vi "PluginManager.vi"() -> ()   [LabVIEW 2018]
doc: "This is the central application/framework that controls module, run scripts, etc"
uses:
  LV_Config_class/Config.lvclass/Config.ctl
  Tree/Controls/Plugins Tree Item Type.ctl
  UserEvents/clUserEventDataType.ctl
  LV_Config_class/Accessors/Read ConfigFilePath.vi
  LV_Config_class/Accessors/Write ConfigFilePath.vi
  <vilib>/Utility/error.llb/Error Cluster From Error Code.vi
  <vilib>/ErrorRing/Error Ring.xnode
  Queue/Queue.lvlib
  <userlib>/NIST/NISTErrorLib/NISTErrorLib.lvlib
  LV_Config_class/Config.lvclass
  <vilib>/Utility/config.llb/NI_LVConfig.lvlib
  Message Queue/Message Queue.lvlib
panel:
  out "found?":bool
  in  "Stop?":bool
  out "OrigPluginTreeTags":string[](array[string])
  out "Plugin Tree Caption":string="Available Plugins"
  in  "btnRunModule":bool
  in  "btnRefresh":bool
  in  "btnLoadUserFiles":bool
  in  "btnConfig":bool
  in  "btnAddToTest":bool
  in  "PluginTree":string(tree)
  in  "Experiment Specific Controls":T1(tab)
  in  "Priority":u8=2
  in  "Severity":string="Abort"
  out "Error Out":errorcluster
  in  "Severity":string
  in  "Priority":u8=2
  in  "Create Error (Test AutoTimeout)":bool
  in  "Error In 2":errorcluster
  in  "btnRunScript":bool
  out "Userfiles Folder":path
  in  "btnSaveINIFiles":bool
  in  "btnDeleteScript":bool
  in  "btnNewScript":bool
  in  "btnScriptHelper":bool
  in  "PluginScript":string
  # "Script Preview and Editor"
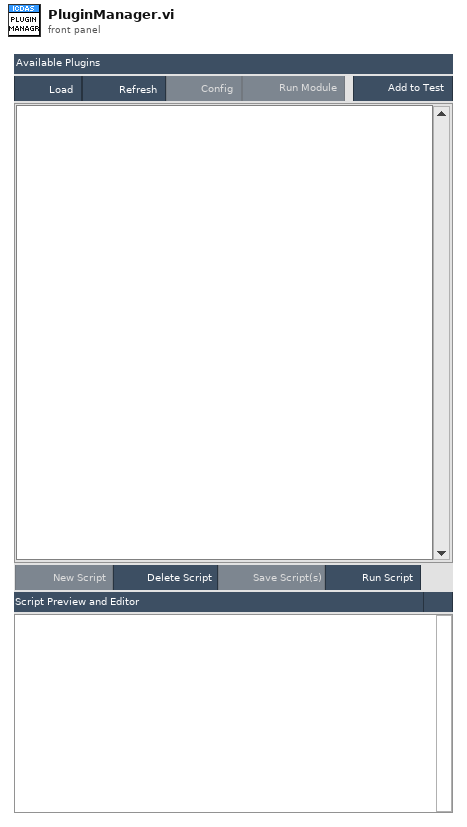
[diagram p1: front panel]
types:
  T1 = enum32{"PV Aging Experiment", "Pacific Power ", "Miscellaneous ", "Errors", "Test AutoTimeout", "Test Python MutliRun"}
  T2 = typedef "ICDASUserEvents.ctl" = cluster{"StopEvent":refnum<user-event>, "RefreshUserEvents":refnum<user-event>, "StatusUpdate":refnum<user-event>, "RunAllScripts":refnum<user-event>, "ShutdownEvent":refnum<user-event>, "TestMgrDidStop":refnum<user-event>, "PluginMgrDidStop":refnum<user-event>}
  T3 = typedef "Message Queue.lvlib/All Message Queues.ctl" = cluster{"UI":refnum<queue>}
  T4 = enum8{"Enabled", "Disabled", "Disabled and Grayed Out"}
  T5 = typedef "Plugins Tree Item Type.ctl" = enum16{"Plugin", "Instrument", "INI File", "INI Script"}
  T6 = typedef "cntlRefs.ctl" = cluster{"rngFGen":refnum<vi>, "rngDigitizer":refnum<vi>, "btnHide":refnum<vi>, "rngInst":refnum<vi>, "PluginTree":refnum<vi>, "TestListboxRef":refnum<vi>, "path.tstFile":refnum<vi>, "cmbxRunningModules":refnum<vi>, "TestDataSubPanel":refnum<vi>, "TestDataCaption":refnum<vi>, "btnPopInOut":refnum<vi>, "PluginMgrQ":refnum<queue>, "TestMgrQ":refnum<queue>, "TestMgrSubPanel":refnum<vi>, "PluginMgrSubPanel":refnum<vi>, "PwrReqHandle":u32, "btnStopOneTest":refnum<vi>, "pathUserfiles":refnum<vi>, "PluginTreeCaption":refnum<vi>, "MainVIRef":refnum<vi>, "btnStatus":refnum<vi>}
  T7 = typedef "NI_LVConfig.lvlib/Config Data RefNum.ctl" = refnum<k1>
  T8 = typedef "Plugin Tree Tag.ctl" = cluster{"ItemType":T5, "Name":string, "Path":path, "Script":string[]}
  T9 = typedef "INIInfo.ctl" = cluster{"Module Name":string, "INI File Name":string, "Class Name":string, "INI File Name Without Extension":string, "Module.Class.INI File Name":string, "Visualization VI Path":path, "Instrument Class Path":path}
  T10 = enum16{"Left Button", "Center Button", "Right Button", "Window Close"}
  T11 = enum32{"Invalid", "Standard", "Closed", "Hidden", "Minimized", "Maximized"}
  T12 = typedef "LVPoint32TypeDef.ctl" = cluster{"Horizontal":i32, "Vertical":i32}
  T13 = typedef "clUserEventDataType.ctl" = cluster{"Data":variant}
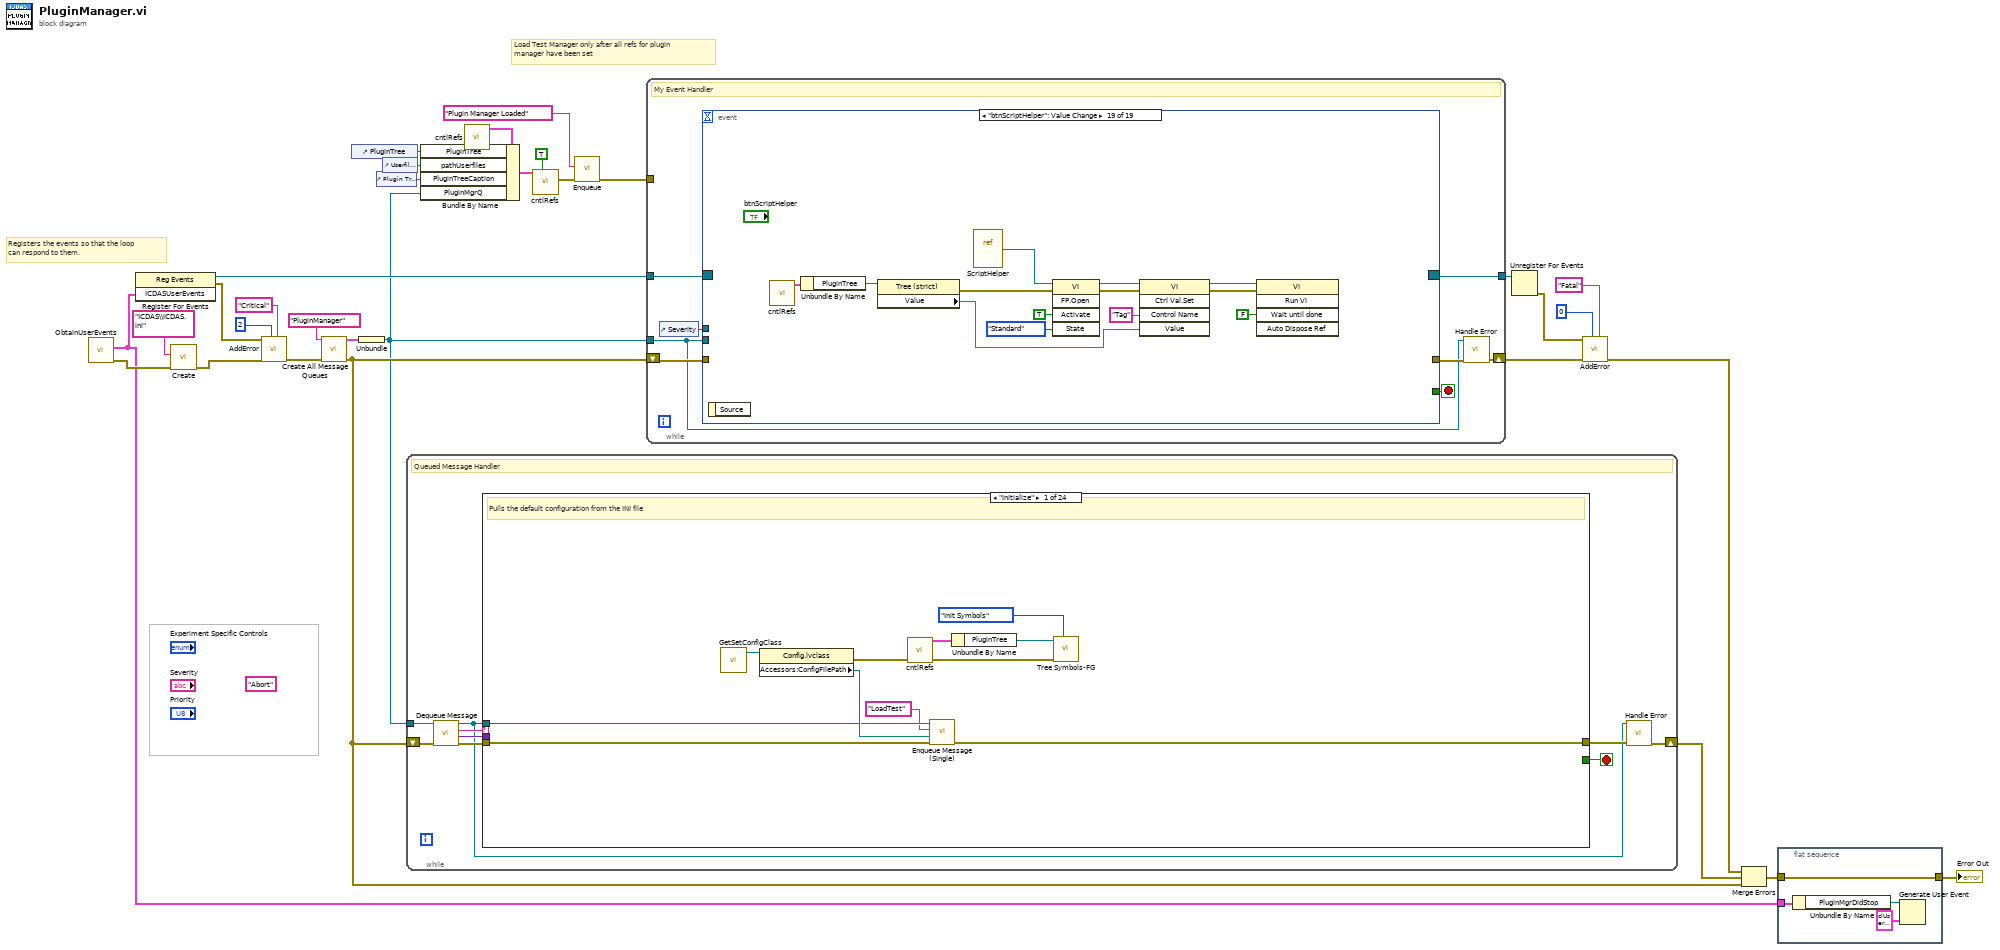
[diagram p0: block diagram]
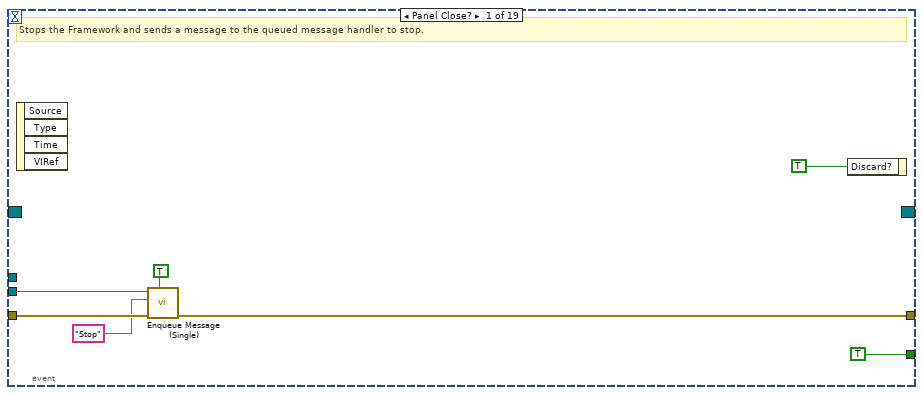
[diagram p2: hidden frame]
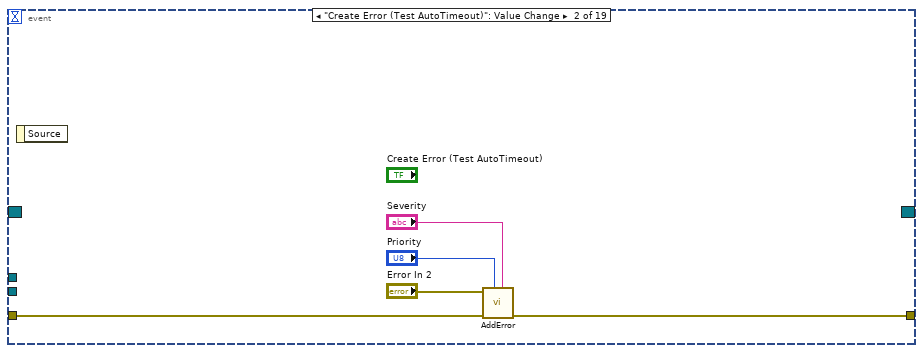
[diagram p3: hidden frame]
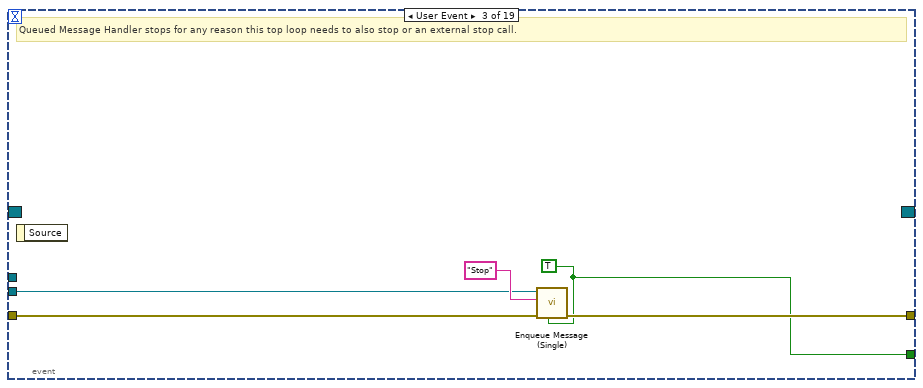
[diagram p4: hidden frame]
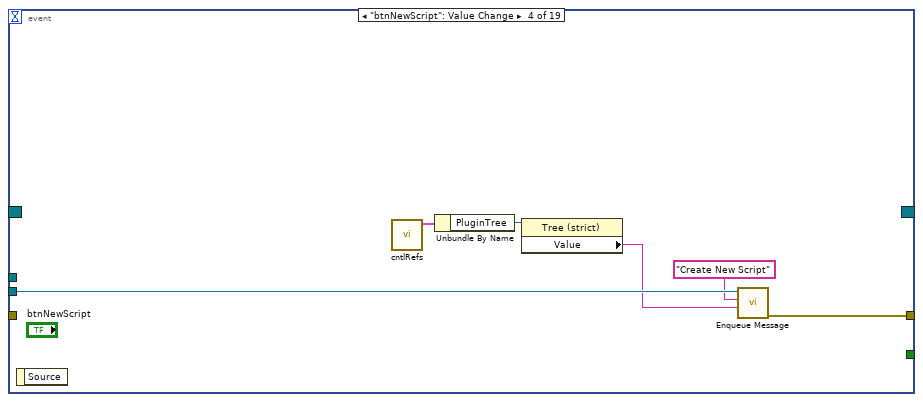
[diagram p5: hidden frame]
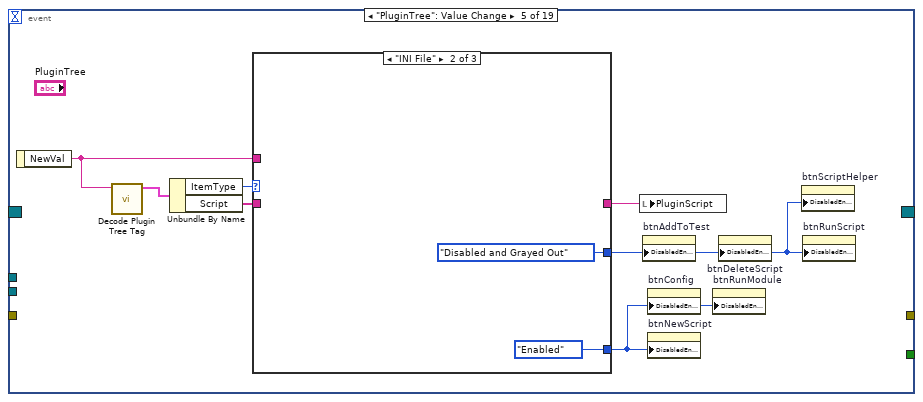
[diagram p6: hidden frame]
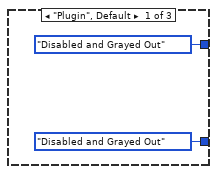
[diagram p7: hidden frame]
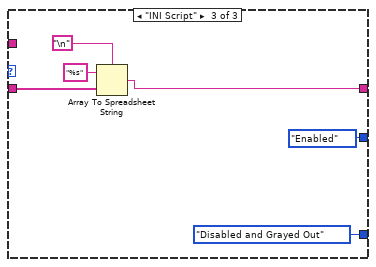
[diagram p8: hidden frame]
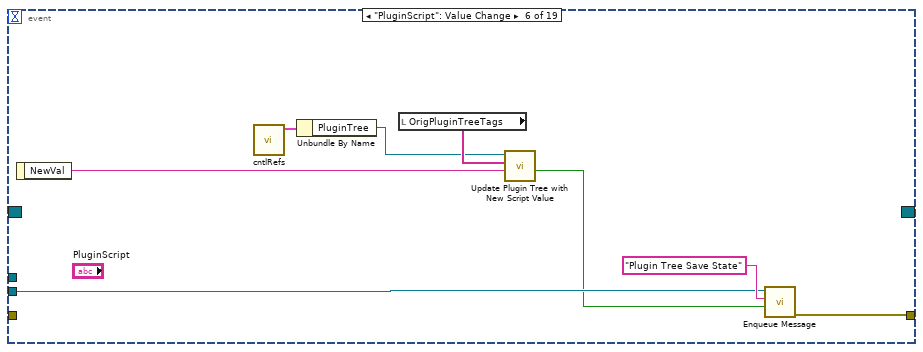
[diagram p9: hidden frame]
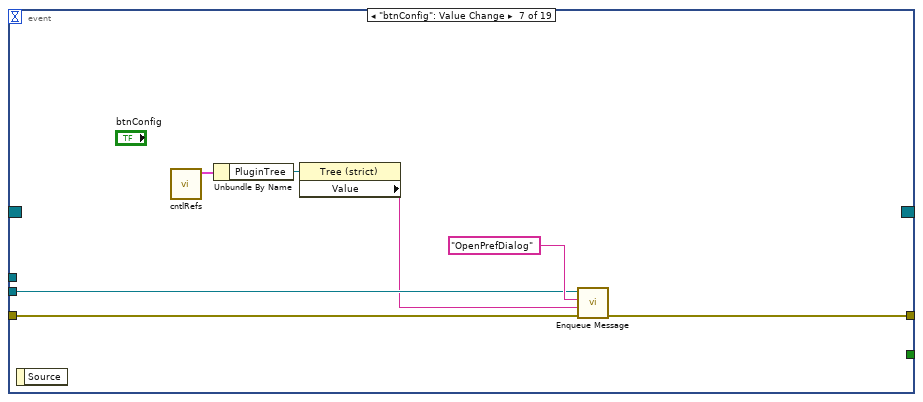
[diagram p10: hidden frame]
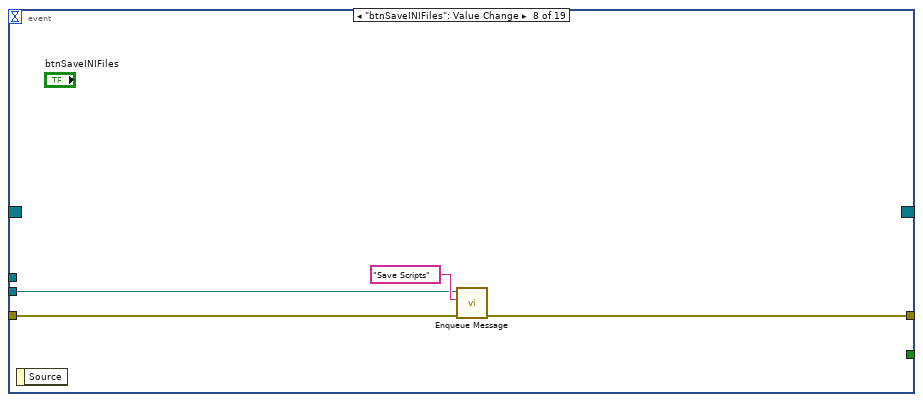
[diagram p11: hidden frame]
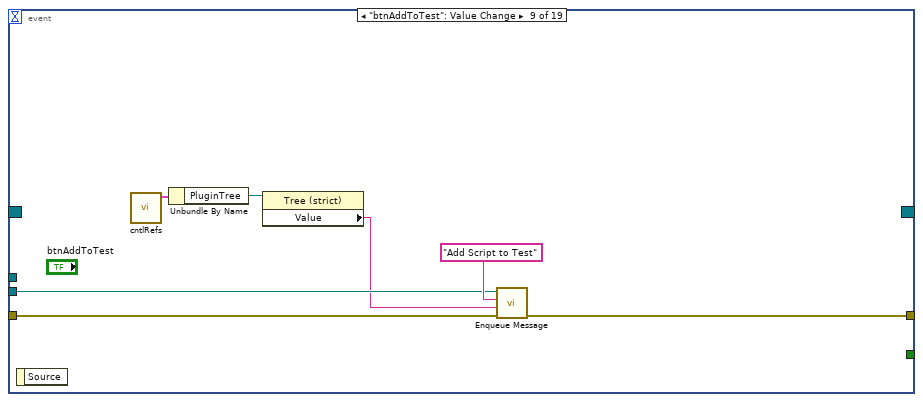
[diagram p12: hidden frame]
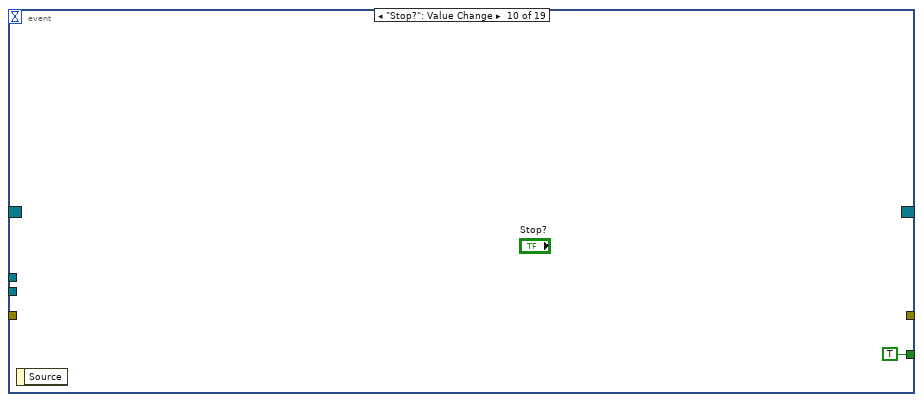
[diagram p13: hidden frame]
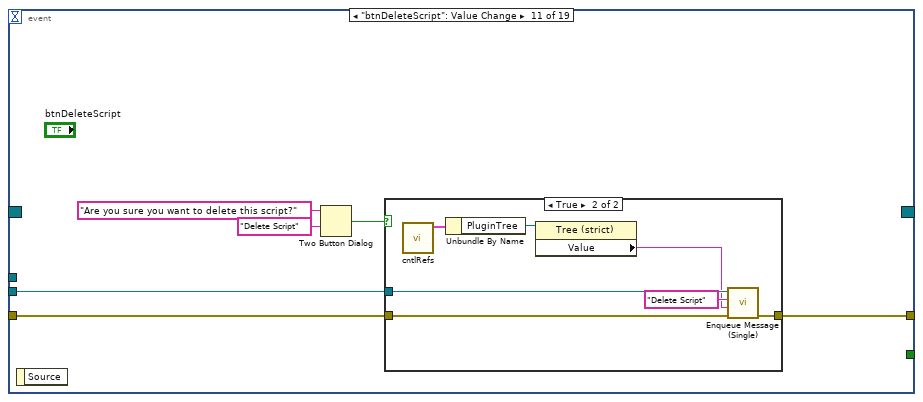
[diagram p14: hidden frame]
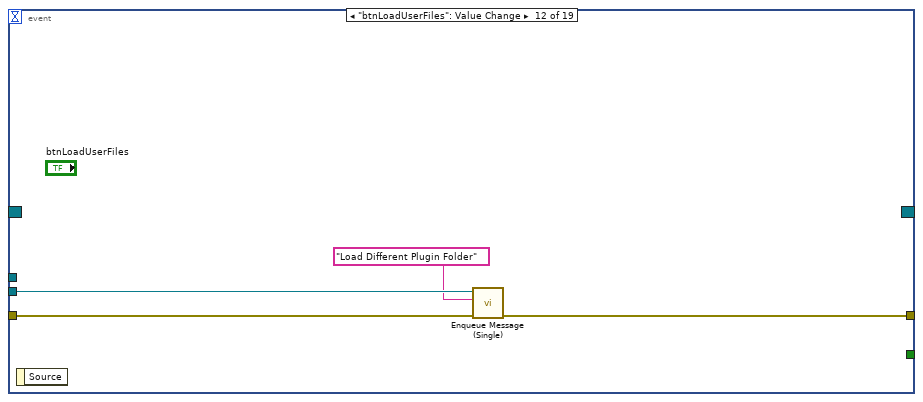
[diagram p16: hidden frame]
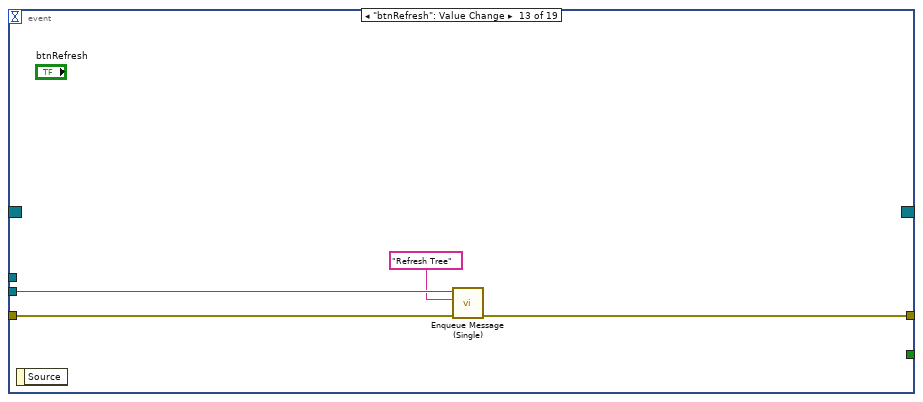
[diagram p17: hidden frame]
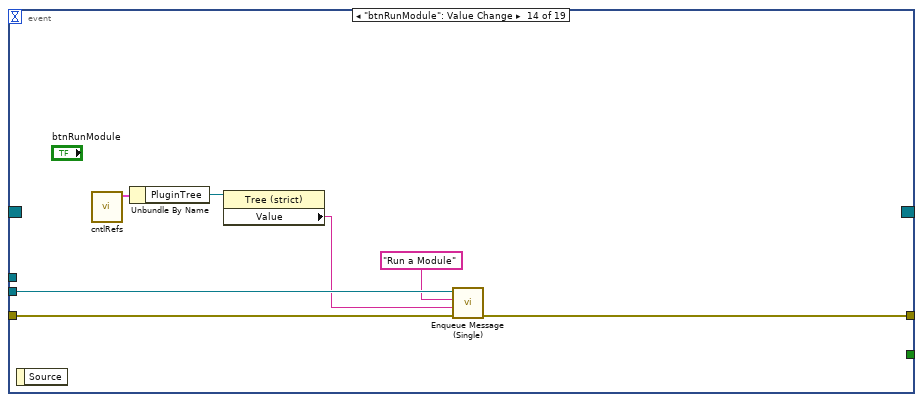
[diagram p18: hidden frame]
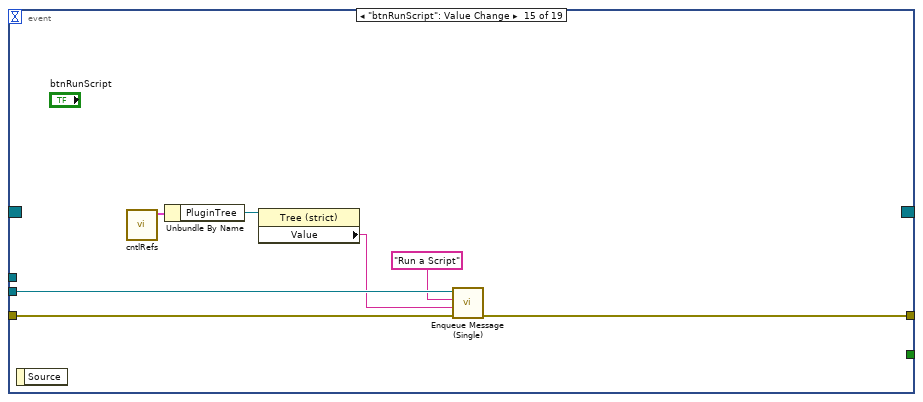
[diagram p19: hidden frame]
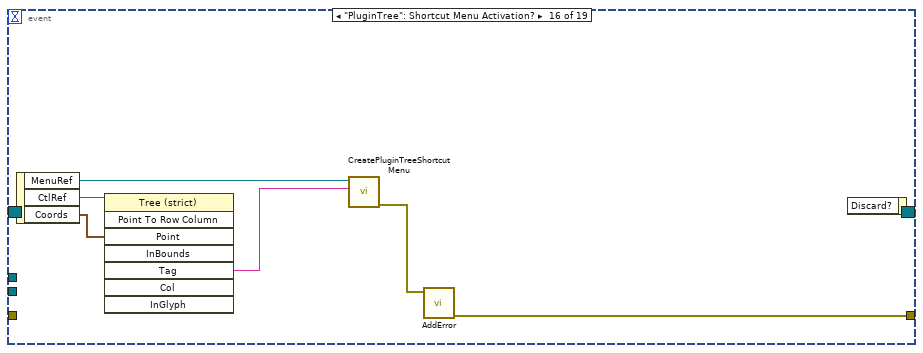
[diagram p20: hidden frame]
diagram:
  (unwired) "Abort" ("Severity")
  # "Load Test Manager only after all refs for plugin\nmanager have been set"
  # "Registers the events so that the loop \ncan respond to them."
  n1 = call "ObtainUserEvents.vi"() -> ("ErrorArray"=w16:errorcluster[], "ICDASUserEvents"=w1:T2)  [unwired: 10 in]
  n2 = register-events(w1) -> (reference out=w31:refnum<event-registration>, error out=w22:errorcluster)  [unwired: 2 in]
  n3 = call "Create.vi"("ErrorArray"=w16, "name or relative path"="ICDAS\\ICDAS.ini") -> ("ErrorArray"=w15:errorcluster[])  [unwired: 8 in, 1 out]
  n4 = call <userlib>:"AddError.vi"("Severity"="Critical", "Priority"=u8 2, "ErrorArray In"=w15, "error in (no error)"=w22) -> ("ErrorArray Out"=w18:errorcluster[])  [unwired: 6 in, 1 out]
  n5 = call "Create All Message Queues.vi"("error in (no error)"=w18, "Queue Name (unnamed)"="PluginManager") -> ("error out"=w9:errorcluster[], "Message Queues out"=w19:T3)  [unwired: 8 in]
  n6 = control-ref of="PluginTree"() -> (w21:refnum<vi>)
  n7 = Unbundle(w19) -> ("UI"=w8:refnum<queue>)
  n8 = control-ref of="Plugin Tree Caption"() -> (w6:refnum<vi>)
  n9 = control-ref of="Userfiles Folder"() -> (w7:refnum<vi>)
  n10 = while {
    shift-right: [w39] -> w27
    shift-left: w9 -> [w34]
    tunnel: w8 -> [w37]
    stop <- w38 stop-if-true
    # "Queued Message Handler"
    n11 = call "Dequeue Message.vi"("error in (no error)"=w34, "Message Queue"=w37) -> ("error out"=w33:errorcluster[], "Message Data"=w36:variant, "Message"=w35:string, "dup Message Queue"=w32:refnum<queue>)  [unwired: 6 in]
    n12 = case shown="\"Initialize\"" w35 {
      selector: w35 -> [_ _ _ _ _ _ w202 _ _ _ _ _ _ _ _ _ _ _ _ _ _ _ _ _]
      tunnel: [w42 w54 w95 w139 w183 w192 w201 w210 w217 w240 w245 w284 w290 w310 w325 w372 w383 w428 w438 w455 w463 w477 w481 w485] -> w40
      tunnel: w33 -> [w44 w53 w100 w138 w178 w196 w200 w210 w223 w240 w247 w284 w302 w314 w319 w374 w384 w428 w437 w454 w464 w477 w481 w485]
      tunnel: [_ _ _ _ _ TRUE _ _ _ _ _ _ _ _ _ _ _ _ _ _ _ _ _ _] -> w38
      tunnel: w36 -> [_ w52 w101 _ w182 _ _ _ w213 w238 w244 w268 w294 w308 _ _ _ _ w432 w449 w461 _ _ _]
      tunnel: w32 -> [w43 w51 w93 w129 w173 w187 _ _ w216 _ w246 _ _ _ w320 w371 w385 _ _ _ _ _ _ _]
      frame "Initialize" {
        # "Pulls the default configuration from the INI file"
        n13 = call "GetSetConfigClass.vi"() -> ("Ref out"=w50:refnum<class "Config.lvclass">)  [unwired: 11 in]
        n14 = property class="Config.lvclass"(reference=w50) -> (error out=w47:errorcluster, "Accessors:ConfigFilePath"=w49:path)  [unwired: 1 in, 1 out]
        n15 = call "cntlRefs.vi"() -> ("cntlRefs"=w46:T6)  [unwired: 10 in, 1 out]
        n16 = call "Enqueue Message (Single).vi"("error in (no error)"=w44, "Message Data"=w49, "Message"="LoadTest", "Message Queue"=w43) -> ("error out"=w42:errorcluster[])  [unwired: 6 in, 1 out]
        n17 = Unbundle By Name(w46) -> ("PluginTree"=w45:refnum<vi>)
        n18 = call "Tree Symbols-FG.vi"("Actions"=enum16{"Init Symbols", "Set Item Symbol"}."Init Symbols", "error in (no error)"=w47, "Tree Ref"=w45) -> ()  [unwired: 5 in, 4 out]
      }
      frame "LoadTest" {
        # "From the default file load the last saved results and updated the controls and indicators"
        n19 = disable-structure shown="Enabled" {
          disable-tunnel: [w87 _] -> w54
          disable-tunnel: w53 -> [w85 _]
          disable-tunnel: w52 -> [w82 w88]
          disable-tunnel: w51 -> [w66 _]
          frame Enabled {
            n20 = call "cntlRefs.vi"() -> ("cntlRefs"=w59:T6)  [unwired: 10 in, 1 out]
            n21 = Unbundle By Name(w59) -> ("pathUserfiles"=w58:refnum<vi>)
            n22 = Variant To Data(type=path "", Variant=w82) -> (data=w83:path, error out=w86:errorcluster)  [unwired: 1 in]
            n23 = call <vilib>:"Open Config Data.vi"("error in (no error)"=w86, "configuration file path"=w83) -> ("error out"=w67:errorcluster, "refnum"=w81:T7)  [unwired: 7 in, 1 out]
            n24 = property class="Path"(reference=w58, error in=w67) -> (error out=w78:errorcluster, "Label.Text"=w79:string)  [unwired: 1 out]
            n25 = call <userlib>:"Read Key (Variant)__ogtk.vi"("section"=w79, "error in (no error)"=w78, "type"="", "key (optional)"=w79, "refnum"=w81) -> ("error out"=w77:errorcluster, "key-value"=w80:variant, "found?"=→"found?":bool)  [unwired: 3 in, 1 out]
            n26 = Variant To Data(error in=w77, type="", Variant=w80) -> (data=w76:string, error out=w73:errorcluster)
            n27 = call <vilib>:"Trim Whitespace.vi"("string"=w76) -> ("trimmed string"=w71:string)  [unwired: 1 in]
            n28 = local read "Severity"() -> (w74:string)
            n29 = local read "Priority"() -> (w75:u8)
            n30 = call <vilib>:"Application Directory.vi"() -> ("Application Directory"=w61:path)
            n31 = Empty String/Path?(string/path=w71) -> (empty?=w70:bool)
            n32 = call <userlib>:"AddError.vi"("Severity"=w74, "Priority"=w75, "ErrorArray In"=w85, "error in (no error)"=w73) -> ("ErrorArray Out"=w64:errorcluster[])  [unwired: 6 in, 1 out]
            n33 = Build Path(base path=w61, name or relative path=w71) -> (appended path=w69:path)
            n34 = Build Path(base path=w61, name or relative path="UserFiles") -> (appended path=w60:path)
            n35 = Select(t=w60, s=w70, f=w69) -> (s? t:f=w68:path)
            n36 = call "Enqueue Defer Panel Updates Message.vi"("error in (no error)"=w64, "Message Queue"=w66) -> ("error out"=w63:errorcluster[], "dup Message Queue"=w65:refnum<queue>)  [unwired: 8 in]
            n37 = call "Enqueue Message (Single).vi"("error in (no error)"=w63, "Message Data"=w68, "Message"="Populate Plugin Tree", "Message Queue"=w65) -> ("error out"=w87:errorcluster[])  [unwired: 6 in, 1 out]
          }
          frame Disabled {
            n38 = disable-structure shown="Disabled" {
              disable-tunnel: w88 -> [w90 _]
              frame Disabled {
                n39 = Variant To Data(type=path "", Variant=w90) -> (data=w91:path, error out=w89:errorcluster)  [unwired: 1 in]
                n40 = call <vilib>:"Open Config Data.vi"("error in (no error)"=w89, "configuration file path"=w91) -> ()  [unwired: 7 in, 3 out]
              }
              frame Enabled {
              }
            }
          }
        }
      }
      frame "Error" {
        n41 = Variant To Data(type=w100, Variant=w101) -> (data=w99:errorcluster[], error out=w94:errorcluster)  [unwired: 1 in]
        n42 = call <userlib>:"ParseErrors.vi"("ErrorArray"=w99) -> ("ErrorArray"=w102:errorcluster[])  [unwired: 8 in, 2 out]
        n43 = for {
          tunnel: w102 -> [w109] mode=indexing
          tunnel: [w112] -> w96 mode=concatenating
          tunnel: w93 -> [w103]
          n44 = call <userlib>:"GeneralHandler.vi"("error in (no error)"=w109) -> ("Severity"=w110:string, "Stop"=w106:bool, "Abort"=w107:bool, "Continue"=w108:bool, "Error Out"=w104:errorcluster)  [unwired: 6 in]
          n45 = Build Array(w108, w107, w106) -> (w105:bool[])
          n46 = Boolean Array To Number(Boolean array=w105) -> (number=w111:u32)
          n47 = case shown="2" w111 {
            tunnel: w110 -> [_ _ _ _]
            tunnel: [_ _ w115 w128] -> w112
            tunnel: w109 -> [_ _ _ _]
            tunnel: w104 -> [_ _ w117 _]
            tunnel: w103 -> [_ _ w114 _]
            frame 0, Default {
              # "No Dialog"
            }
            frame 1 {
              # "Continue"
            }
            frame 2 {
              # "Abort Button Pressed"
              n48 = Flush Queue(queue=w114, error in (no error)=w117) -> (queue out=w113:refnum<queue>, error out=w120:errorcluster)  [unwired: 1 out]
              n49 = call <userlib>:"AddError.vi"("Severity"="Critical", "Priority"=u8 1, "error in (no error)"=w120) -> ("ErrorArray Out"=w116:errorcluster[])  [unwired: 7 in, 1 out]
              n50 = disable-structure shown="Disabled" {
                disable-tunnel: w116 -> [w124 w127]
                disable-tunnel: [w123 w127] -> w115
                disable-tunnel: w113 -> [w121 _]
                frame Disabled {
                  n51 = To Variant(anything="*AbortScript" ("Message")) -> (Variant=w125:variant)
                  n52 = call-poly "Enqueue Message.vi"("error in (no error)"=w124, "Message Data"=w125, "Message"="RunOneTest", "Message Queue"=w121) -> ("error out"=w123:errorcluster[])  [unwired: 6 in, 1 out]
                }
                frame Enabled {
                }
              }
            }
            frame 4 {
              # "Stop this application"
              n53 = call "StopEvent.vi"() -> ("ErrorArray"=w128:errorcluster[])  [unwired: 11 in]
            }
          }
        }
        n54 = call <userlib>:"AddError.vi"("Severity"="Fatal", "Priority"=u8 0, "ErrorArray In"=w96, "error in (no error)"=w94) -> ("ErrorArray Out"=w95:errorcluster[])  [unwired: 6 in, 1 out]
      }
      frame "Stop" {
        n55 = disable-structure shown="Enabled" {
          disable-tunnel: [w158 FALSE ("T button?")] -> w134
          frame Disabled {
            n56 = Two Button Dialog(message="Save Application configuration to a new location?") -> (T button?=w158:bool)  [unwired: 2 in]
          }
          frame Enabled {
          }
        }
        n57 = call "GetSetConfigClass.vi"() -> ("Ref out"=w142:refnum<class "Config.lvclass">)  [unwired: 11 in]
        n58 = property class="Config.lvclass"(reference=w142) -> (reference out=w132:refnum<class "Config.lvclass">, error out=w135:errorcluster, "Accessors:ConfigFilePath"=w136:path)  [unwired: 1 in]
        n59 = case shown="True" w134 {
          tunnel: w136 -> [w143 w154]
          tunnel: w135 -> [w144 w153]
          tunnel: [w144 w145] -> w133
          tunnel: w132 -> [_ w149]
          tunnel: [w143 w146] -> w131
          frame False {
          }
          frame True {
            n60 = call "FileDialog.vi"("Error In"=w153, "File Path Control In"=w154) -> ("Error Out"=w151:errorcluster, "Valid File Path?"=w148:bool, "File Path Control Out"=w147:path)  [unwired: 7 in]
            n61 = Select(t=w147, s=w148, f=w154) -> (s? t:f=w152:path)
            n62 = property class="Config.lvclass"(reference=w149, error in=w151, "Accessors:ConfigFilePath"=w152) -> (reference out=w150:refnum<class "Config.lvclass">, error out=w145:errorcluster, "Accessors:ConfigFilePath"=w146:path)
            n63 = flat-sequence {
              tunnel: w150 -> [w157]
              tunnel: w145 -> [_]
              frame #0 {
                n64 = Two Button Dialog(message="Update configuration file path") -> (T button?=w156:bool)  [unwired: 2 in]
                n65 = call "GetSetConfigClass.vi"("Set (f)"=w156, "Ref in"=w157) -> ()  [unwired: 9 in, 1 out]
              }
            }
          }
        }
        n66 = local read "Severity"() -> (w130:string)
        n67 = call-poly "Enqueue Message.vi"("error in (no error)"=w138, "Message Data"=w131, "Message"="SaveTest", "Message Queue"=w129) -> ("error out"=w137:errorcluster[])  [unwired: 6 in, 1 out]
        n68 = call <userlib>:"AddError.vi"("Severity"=w130, "Priority"=u8 0, "ErrorArray In"=w137, "error in (no error)"=w133) -> ("ErrorArray Out"=w139:errorcluster[])  [unwired: 6 in, 1 out]
      }
      frame "SaveTest" {
        # "saves the state of the controls and indicators into an INI file"
        n69 = Variant To Data(type=path "", Variant=w182) -> (data=w177:path, error out=w181:errorcluster)  [unwired: 1 in]
        n70 = call <vilib>:"Open Config Data.vi"("error in (no error)"=w181, "configuration file path"=w177) -> ("error out"=w180:errorcluster, "refnum"=w176:T7)  [unwired: 7 in, 1 out]
        n71 = call <userlib>:"AddError.vi"("ErrorArray In"=w178, "error in (no error)"=w180) -> ("ErrorArray Out"=w179:errorcluster[])  [unwired: 8 in, 1 out]
        n72 = call "cntlRefs.vi"() -> ("cntlRefs"=w174:T6)  [unwired: 10 in, 1 out]
        n73 = Unbundle By Name(w174) -> ("pathUserfiles"=w170:refnum<vi>)
        n74 = property class="Path"(reference=w170) -> (error out=w166:errorcluster, "Label.Text"=w167:string, "Value"=w165:path)  [unwired: 1 in, 1 out]
        n75 = call "ConvertAbsolutePathToRelative.vi"("Absolute Path"=w165) -> ("RelativePath"=w164:string)  [unwired: 10 in]
        n76 = call <userlib>:"Write Key (Variant)__ogtk.vi"("section"=w167, "error in (no error)"=w166, "key-value"=w164, "key (optional)"=w167, "refnum"=w176) -> ("error out"=w163:errorcluster, "refnum out"=w161:T7)  [unwired: 5 in]
        n77 = call <vilib>:"Close Config Data.vi"("error in (no error)"=w163, "refnum"=w161) -> ("error out"=w162:errorcluster)  [unwired: 8 in, 1 out]
        n78 = call <userlib>:"AddError.vi"("Severity"="Abort", "Priority"=u8 3, "ErrorArray In"=w179, "error in (no error)"=w162) -> ("ErrorArray Out"=w171:errorcluster[])  [unwired: 6 in, 1 out]
        n79 = call-poly "Enqueue Message.vi"("error in (no error)"=w171, "Message"="End", "Message Queue"=w173) -> ("error out"=w183:errorcluster[])  [unwired: 7 in, 1 out]
      }
      frame "End" {
        n80 = call "cntlRefs.vi"() -> ("cntlRefs"=w191:T6)  [unwired: 10 in, 1 out]
        n81 = Unbundle By Name(w191) -> ("PluginTree"=w190:refnum<vi>)
        n82 = local write "PluginScript"("") -> ()
        n83 = invoke class="Tree (strict)" method="Edit Tree Items.Delete"(reference=w190, "Delete Children"=TRUE ("Delete Children?")) -> ()  [unwired: 3 in, 5 out]
        n84 = Release Queue(queue=w187, force destroy? (F)=TRUE) -> (error out=w186:errorcluster)  [unwired: 1 in, 2 out]
        n85 = property on="Stop?" class="Bool (strict)"("Val(Sgnl)"=TRUE ("Value (Signaling)")) -> ()  [unwired: 2 in, 2 out]
        n86 = call <userlib>:"AddError.vi"("Severity"="Abort", "Priority"=u8 3, "ErrorArray In"=w196, "error in (no error)"=w186) -> ("ErrorArray Out"=w192:errorcluster[])  [unwired: 6 in, 1 out]
      }
      frame Default {
        n87 = xnode "Error Ring"("parameter 0"=w202) -> ("error out"=w197:errorcluster)
        n88 = call <userlib>:"AddError.vi"("Severity"="Inform", "Priority"=u8 5, "ErrorArray In"=w200, "error in (no error)"=w197) -> ("ErrorArray Out"=w201:errorcluster[])  [unwired: 6 in, 1 out]
      }
      frame "----Plugin Setup----" {
      }
      frame "Populate Plugin Tree" {
        # "Clear tree value and script control"
        n89 = Variant To Data(type=path "", Variant=w213) -> (data=w211:path)  [unwired: 1 in, 1 out]
        "Userfiles Folder" <- w211
        n90 = call "cntlRefs.vi"() -> ("cntlRefs"=w215:T6)  [unwired: 10 in, 1 out]
        n91 = Unbundle By Name(w215) -> ("PluginTree"=w214:refnum<vi>)
        n92 = call "Populate Plugin Tree.vi"("ErrorArray In"=w223, "Userfiles Directory"=w211, "PluginTreeRef"=w214) -> ("ErrorArray Out"=w218:errorcluster[], "All Tags"=→"OrigPluginTreeTags":string[], "Tree Ref out"=w225:refnum<vi>)  [unwired: 5 in, 1 out]
        n93 = property class="Tree (strict)"(reference=w225, "Val(Sgnl)"="") -> ()  [unwired: 1 in, 2 out]
        n94 = call "Enqueue Message (Single).vi"("error in (no error)"=w218, "Message Data"=FALSE, "Message"="Plugin Tree Save State", "Message Queue"=w216) -> ("error out"=w222:errorcluster[], "dup Message Queue"=w221:refnum<queue>)  [unwired: 6 in]
        n95 = call "Enqueue Update Panel Message.vi"("error in (no error)"=w222, "Message Queue"=w221) -> ("error out"=w217:errorcluster[])  [unwired: 8 in, 1 out]
      }
      frame "Plugin Tree Save State" {
        n96 = Variant To Data(type=FALSE, Variant=w238) -> (data=w234:bool)  [unwired: 1 in, 1 out]
        n97 = local read "Userfiles Folder"() -> (w230:path)
        n98 = call "ConvertAbsolutePathToRelative.vi"("Absolute Path"=w230) -> ("RelativePath"=w227:string)  [unwired: 10 in]
        n99 = Format Into String(format string="Available Plugins - %s" ("Message"), w227) -> (resulting string=w228:string)  [unwired: 2 in, 1 out]
        n100 = Concatenate Strings(w228, "*" ("string")) -> (w236:string)
        n101 = Select(t=w236, s=w234, f=w228) -> (s? t:f=→"Plugin Tree Caption":string)
        n102 = Select(t=T4."Enabled" ("Disabled"), s=w234, f=T4."Disabled and Grayed Out" ("Disabled")) -> (s? t:f=w232:T4)
        n103 = property on="btnSaveINIFiles" class="Bool"("DisabledEnum"=w232) -> ()  [unwired: 2 in, 2 out]
      }
      frame "Create New Script" {
        n104 = Variant To Data(type="", Variant=w244) -> (data=w242:string, error out=w241:errorcluster)  [unwired: 1 in]
        n105 = call "cntlRefs.vi"() -> ("cntlRefs"=w252:T6)  [unwired: 10 in, 1 out]
        n106 = call "Decode Plugin Tree Tag.vi"("error in (no error)"=w241, "Tag"=w242) -> ("error out"=w250:errorcluster, "Plugin Tree Tag"=w248:T8)  [unwired: 8 in]
        n107 = Unbundle By Name(w252) -> ("PluginTree"=w251:refnum<vi>)
        n108 = Unbundle By Name(w248) -> ("ItemType"=w249:T5)
        n109 = case shown="\"INI File\"" w249 {
          tunnel: w251 -> [_ w261]
          tunnel: w250 -> [_ w259]
          tunnel: w242 -> [_ w260]
          tunnel: w246 -> [_ w256]
          tunnel: [w253 w255] -> w245
          tunnel: w247 -> [w253 w254]
          frame "Plugin", Default {
          }
          frame "INI File" {
            n110 = call "Add New Script to Tree.vi"("error in (no error)"=w259, "Value"=w260, "TreeControl in"=w261) -> ("error out"=w257:errorcluster, "Cancelled?"=w258:bool)  [unwired: 7 in]
            n111 = case shown="False" w258 {
              tunnel: w257 -> [_ _]
              tunnel: w256 -> [w264 _]
              tunnel: [w263 _] -> w255
              tunnel: w254 -> [w262 _]
              frame False {
                n112 = call-poly "Enqueue Message.vi"("error in (no error)"=w262, "Message Data"=TRUE, "Message"="Plugin Tree Save State", "Message Queue"=w264) -> ("error out"=w263:errorcluster[])  [unwired: 6 in, 1 out]
              }
              frame True {
              }
            }
          }
        }
      }
      frame "Delete Script" {
        n113 = Variant To Data(type="", Variant=w268) -> (data=w267:string)  [unwired: 1 in, 1 out]
        n114 = call "cntlRefs.vi"() -> ("cntlRefs"=w283:T6)  [unwired: 10 in, 1 out]
        n115 = Unbundle By Name(w283) -> ("PluginTree"=w282:refnum<vi>)
        n116 = invoke class="Tree (strict)" method="Edit Tree Items.Delete"(reference=w282, "tag"=w267, "Delete Children"=TRUE ("Delete Children?")) -> (error out=w271:errorcluster)  [unwired: 2 in, 4 out]
        n117 = call "Decode Plugin Tree Tag.vi"("error in (no error)"=w271, "Tag"=w267) -> ("error out"=w273:errorcluster, "Plugin Tree Tag"=w281:T8)  [unwired: 8 in]
        n118 = Unbundle By Name(w281) -> ("Name"=w275:string, "Path"=w280:path)
        n119 = call <vilib>:"Open Config Data.vi"("error in (no error)"=w273, "configuration file path"=w280) -> ("error out"=w278:errorcluster, "refnum"=w279:T7)  [unwired: 7 in, 1 out]
        n120 = Concatenate Strings("*" ("string"), w275) -> (w270:string)
        n121 = call <vilib>:"Remove Section.vi"("section"=w270, "error in (no error)"=w278, "refnum"=w279) -> ("error out"=w276:errorcluster, "refnum out"=w277:T7)  [unwired: 6 in, 1 out]
        n122 = call <vilib>:"Close Config Data.vi"("error in (no error)"=w276, "refnum"=w277) -> ()  [unwired: 8 in, 2 out]
      }
      frame "OpenPrefDialog" {
        # "Get module name from INI File Path"
        # "runs the SSM using a set script"
        n123 = call "cntlRefs.vi"() -> ("cntlRefs"=w288:T6)  [unwired: 10 in, 1 out]
        n124 = Unbundle By Name(w288) -> ("MainVIRef"=w287:refnum<vi>)
        n125 = call <vilib>:"Set Busy.vi"("VI reference (current VI)"=w287) -> ("error out"=w291:errorcluster)  [unwired: 9 in, 1 out]
        n126 = Variant To Data(error in=w291, type="", Variant=w294) -> (data=w293:string, error out=w292:errorcluster)
        n127 = call "Decode Plugin Tree Tag.vi"("error in (no error)"=w292, "Tag"=w293) -> ("error out"=w297:errorcluster, "Plugin Tree Tag"=w301:T8)  [unwired: 8 in]
        n128 = Unbundle By Name(w301) -> ("Path"=w300:path)
        n129 = call <userlib>:"AddError.vi"("Severity"="Inform", "Priority"=u8 2, "ErrorArray In"=w302, "error in (no error)"=w297) -> ("ErrorArray Out"=w296:errorcluster[])  [unwired: 6 in, 1 out]
        n130 = call "ExtractINIInfo.vi"("INI File Path"=w300) -> ("INI Info"=w286:T9)  [unwired: 8 in, 2 out]
        n131 = Unbundle By Name(w286) -> ("Module.Class.INI File Name"=w285:string)
        n132 = call "Load PrefDialog For an INI File.vi"("Error Array In"=w296, "PathToPluginINI"=w300, "Plugin Name"=w285) -> ("ErrorArray Out"=w290:errorcluster[])  [unwired: 8 in]
        n133 = Index Array(array=w290) -> (element=w289:errorcluster)  [unwired: 1 in]
        n134 = call <vilib>:"Unset Busy.vi"("error in (no error)"=w289, "VI reference (current VI)"=w287) -> ()  [unwired: 9 in, 1 out]
      }
      frame "Open in Editor" {
        # "Get module name from INI File Path"
        # "runs the SSM using a set script"
        n135 = Variant To Data(type="", Variant=w308) -> (data=w307:string, error out=w306:errorcluster)  [unwired: 1 in]
        n136 = call "Decode Plugin Tree Tag.vi"("error in (no error)"=w306, "Tag"=w307) -> ("error out"=w304:errorcluster, "Plugin Tree Tag"=w313:T8)  [unwired: 8 in]
        n137 = Unbundle By Name(w313) -> ("Path"=w305:path)
        n138 = call <vilib>:"Open a Document on Disk.vi"("error in (no error)"=w304, "document path"=w305) -> ("error out"=w303:errorcluster)  [unwired: 5 in]
        n139 = call <userlib>:"AddError.vi"("Severity"="Inform", "Priority"=u8 2, "ErrorArray In"=w314, "error in (no error)"=w303) -> ("ErrorArray Out"=w310:errorcluster[])  [unwired: 6 in, 1 out]
      }
      frame "Load Different Plugin Folder" {
        n140 = local read "Plugin Tree Caption"() -> (w324:string)
        n141 = Match Pattern(string=w324, regular expression="*") -> (offset past match=w322:i32)  [unwired: 1 in, 3 out]
        n142 = Greater Than 0?(x=w322) -> (x > 0?=w316:bool)
        n143 = case shown="True" w316 {
          tunnel: "There are unsaved changes in the plugin structure.Please select what you would like to do next." ("message") -> [_ w339]
          tunnel: w320 -> [w327 w333]
          tunnel: w319 -> [w326 w332]
          tunnel: [TRUE ("Allow user to close window? (TRUE)") w331] -> w321
          tunnel: [w327 w330] -> w318
          tunnel: [w326 w329] -> w317
          frame False {
          }
          frame True {
            n144 = call <vilib>:"Three Button Dialog.vi"("Allow user to close window? (TRUE)"=FALSE, "Justify Message (Left)"=enum16{"Left", "Center", "Right"}."Center", "Center Button Text (\"No\")"="Discard Changes & Load" ("Left Button Text (\"Yes\")"), "Left Button Text (\"Yes\")"="Save Changes & Load" ("Left Button Text (\"Yes\")"), "message"=w339) -> ("Which Button?"=w334:T10)  [unwired: 6 in]
            n145 = case shown="\"Left Button\"" w334 {
              tunnel: w333 -> [w343 w347 w350]
              tunnel: w332 -> [w344 w346 w349]
              tunnel: [TRUE ("Allow user to close window? (TRUE)") TRUE ("Allow user to close window? (TRUE)") FALSE ("Allow user to close window? (TRUE)")] -> w331
              tunnel: [w341 w347 w350] -> w330
              tunnel: [w340 w346 w349] -> w329
              frame "Left Button" {
                n146 = call "Enqueue Message (Single).vi"("error in (no error)"=w344, "Message"="Save Scripts", "Message Queue"=w343) -> ("error out"=w340:errorcluster[], "dup Message Queue"=w341:refnum<queue>)  [unwired: 7 in]
              }
              frame "Center Button" {
              }
              frame "Right Button", Default {
              }
            }
          }
        }
        n147 = case shown="True" w321 {
          tunnel: w317 -> [w352 w356]
          tunnel: w318 -> [_ w355]
          tunnel: [w352 w354] -> w325
          frame False {
          }
          frame True {
            n148 = call <vilib>:"Application Directory.vi"() -> ("Application Directory"=w359:path)
            n149 = call "File Dialog"("start path"=w359, "prompt"="Navigate into \"UserFiles\" folder and press \"Select Folder\" button to load...") -> ("selected path"=w353:path, "cancelled"=w357:bool)  [unwired: 10 in, 2 out]
            n150 = case shown="False" w357 {
              tunnel: w356 -> [w362 w367]
              tunnel: w355 -> [w363 _]
              tunnel: [w365 w367] -> w354
              tunnel: w353 -> [w364 _]
              frame False {
                n151 = call "Enqueue Defer Panel Updates Message.vi"("error in (no error)"=w362, "Message Queue"=w363) -> ("error out"=w360:errorcluster[], "dup Message Queue"=w361:refnum<queue>)  [unwired: 8 in]
                n152 = call "Enqueue Message (Single).vi"("error in (no error)"=w360, "Message Data"=w364, "Message"="Populate Plugin Tree", "Message Queue"=w361) -> ("error out"=w365:errorcluster[])  [unwired: 6 in, 1 out]
              }
              frame True {
              }
            }
          }
        }
      }
      frame "Save Scripts" {
        # "After saving the new configuratin, replace the Original Tags\nAND\nRefresh test scrip previoew in Test Manager"
        # "Set tree state to FALSE or already saved"
        n153 = call "cntlRefs.vi"() -> ("cntlRefs"=w380:T6)  [unwired: 10 in, 1 out]
        n154 = Unbundle By Name(w380) -> ("TestMgrQ"=w370:refnum<queue>, "PluginTree"=w379:refnum<vi>)
        n155 = call "Save Plugin Scripts.vi"("TreeControl in"=w379) -> ("error out"=w378:errorcluster, "New Tags After Save"=w377:string[])  [unwired: 8 in, 1 out]
        n156 = property on="OrigPluginTreeTags" class="Arr (strict)"(error in=w378, "Value"=w377) -> (error out=w368:errorcluster)  [unwired: 1 in, 1 out]
        n157 = call-poly "Enqueue Message.vi"("Message"="Refresh Test Script", "Message Queue"=w370) -> ()  [unwired: 8 in, 2 out]
        n158 = call <userlib>:"AddError.vi"("Severity"="Inform", "Priority"=u8 2, "ErrorArray In"=w374, "error in (no error)"=w368) -> ("ErrorArray Out"=w373:errorcluster[])  [unwired: 6 in, 1 out]
        n159 = call-poly "Enqueue Message.vi"("error in (no error)"=w373, "Message Data"=FALSE, "Message"="Plugin Tree Save State", "Message Queue"=w371) -> ("error out"=w372:errorcluster[])  [unwired: 6 in, 1 out]
      }
      frame "Refresh Tree" {
        n160 = local read "Plugin Tree Caption"() -> (w388:string)
        n161 = Match Pattern(string=w388, regular expression="*") -> (offset past match=w386:i32)  [unwired: 1 in, 3 out]
        n162 = Greater Than 0?(x=w386) -> (x > 0?=w389:bool)
        n163 = case shown="True" w389 {
          tunnel: "There are unsaved changes in the plugin structure.Please select what you would like to do next." ("message") -> [_ w407]
          tunnel: w385 -> [w395 w401]
          tunnel: w384 -> [w394 w400]
          tunnel: [TRUE ("Allow user to close window? (TRUE)") w399] -> w391
          tunnel: [w395 w398] -> w392
          tunnel: [w394 w397] -> w393
          frame False {
          }
          frame True {
            n164 = call <vilib>:"Three Button Dialog.vi"("Allow user to close window? (TRUE)"=FALSE, "Justify Message (Left)"=enum16{"Left", "Center", "Right"}."Center", "Center Button Text (\"No\")"="Discard Changes & Refresh" ("Left Button Text (\"Yes\")"), "Left Button Text (\"Yes\")"="Save Changes & Refresh" ("Left Button Text (\"Yes\")"), "message"=w407) -> ("Which Button?"=w402:T10)  [unwired: 6 in]
            n165 = case shown="\"Left Button\"" w402 {
              tunnel: w401 -> [w411 w415 w418]
              tunnel: w400 -> [w412 w414 w417]
              tunnel: [TRUE ("Allow user to close window? (TRUE)") TRUE ("Allow user to close window? (TRUE)") FALSE ("Allow user to close window? (TRUE)")] -> w399
              tunnel: [w409 w415 w418] -> w398
              tunnel: [w408 w414 w417] -> w397
              frame "Left Button" {
                n166 = call "Enqueue Message (Single).vi"("error in (no error)"=w412, "Message"="Save Scripts", "Message Queue"=w411) -> ("error out"=w408:errorcluster[], "dup Message Queue"=w409:refnum<queue>)  [unwired: 7 in]
              }
              frame "Center Button" {
              }
              frame "Right Button", Default {
              }
            }
          }
        }
        n167 = case shown="True" w391 {
          tunnel: w392 -> [_ w422]
          tunnel: w393 -> [w420 w423]
          tunnel: [w420 w426] -> w383
          frame False {
          }
          frame True {
            n168 = local read "Userfiles Folder"() -> (w425:path)
            n169 = call "Enqueue Defer Panel Updates Message.vi"("error in (no error)"=w423, "Message Queue"=w422) -> ("error out"=w421:errorcluster[], "dup Message Queue"=w424:refnum<queue>)  [unwired: 8 in]
            n170 = call "Enqueue Message (Single).vi"("error in (no error)"=w421, "Message Data"=w425, "Message"="Populate Plugin Tree", "Message Queue"=w424) -> ("error out"=w426:errorcluster[])  [unwired: 6 in, 1 out]
          }
        }
      }
      frame "----Commands to TestManager----" {
      }
      frame "Run a Module" {
        # "Create a dummy script tag for the INI file"
        n171 = Variant To Data(type="", Variant=w432) -> (data=w430:string, error out=w429:errorcluster)  [unwired: 1 in]
        n172 = call "Decode Plugin Tree Tag.vi"("error in (no error)"=w429, "Tag"=w430) -> ("error out"=w440:errorcluster, "Plugin Tree Tag"=w444:T8)  [unwired: 8 in]
        n173 = call "cntlRefs.vi"() -> ("cntlRefs"=w439:T6)  [unwired: 10 in, 1 out]
        n174 = Unbundle By Name(w439) -> ("TestMgrQ"=w435:refnum<queue>)
        n175 = Unbundle By Name(w444) -> ("Path"=w442:path)
        n176 = call "Create Plugin Tree Tag.vi"("ItemType"=Plugins_Tree_Item_Type."INI Script", "error in (no error)"=w440, "Name"="Run Module" ("Message"), "VISA Resource"=w442) -> ("Tag"=w434:string)  [unwired: 5 in, 2 out]
        n177 = Build Array(w434) -> (w433:string[])
        n178 = call-poly "Enqueue Message.vi"("error in (no error)"=w437, "Message Data"=w433, "Message"="RunOneTest", "Message Queue"=w435) -> ("error out"=w438:errorcluster[])  [unwired: 6 in, 1 out]
      }
      frame "Run a Script" {
        # "Run the selected script"
        n179 = Variant To Data(type="", Variant=w449) -> (data=w448:string, error out=w446:errorcluster)  [unwired: 1 in]
        n180 = call <userlib>:"AddError.vi"("Severity"="Inform", "ErrorArray In"=w454, "error in (no error)"=w446) -> ("ErrorArray Out"=w447:errorcluster[])  [unwired: 7 in, 1 out]
        n181 = call "cntlRefs.vi"() -> ("cntlRefs"=w456:T6)  [unwired: 10 in, 1 out]
        n182 = Unbundle By Name(w456) -> ("TestMgrQ"=w452:refnum<queue>)
        n183 = Build Array(w448) -> (w451:string[])
        n184 = call-poly "Enqueue Message.vi"("error in (no error)"=w447, "Message Data"=w451, "Message"="RunOneTest", "Message Queue"=w452) -> ("error out"=w455:errorcluster[])  [unwired: 6 in, 1 out]
      }
      frame "Add Script to Test" {
        n185 = Variant To Data(type="", Variant=w461) -> (data=w460:string, error out=w458:errorcluster)  [unwired: 1 in]
        n186 = call <userlib>:"AddError.vi"("Severity"="Inform", "ErrorArray In"=w464, "error in (no error)"=w458) -> ("ErrorArray Out"=w459:errorcluster[])  [unwired: 7 in, 1 out]
        n187 = local read "Plugin Tree Caption"() -> (w465:string)
        n188 = Match Pattern(string=w465, regular expression="*") -> (offset past match=w468:i32)  [unwired: 1 in, 3 out]
        n189 = Less Than 0?(x=w468) -> (x < 0?=w467:bool)
        n190 = case shown="True" w467 {
          tunnel: w459 -> [w470 w476]
          tunnel: [w470 w475] -> w463
          tunnel: w460 -> [_ w471]
          frame False {
            n191 = One Button Dialog(message="Please save plugins before adding to Test Configuration.") -> ()  [unwired: 1 in, 1 out]
          }
          frame True {
            # "Send message to Test Manager to add script to test tree"
            n192 = call "cntlRefs.vi"() -> ("cntlRefs"=w474:T6)  [unwired: 10 in, 1 out]
            n193 = Unbundle By Name(w474) -> ("TestMgrQ"=w473:refnum<queue>)
            n194 = call-poly "Enqueue Message.vi"("error in (no error)"=w476, "Message Data"=w471, "Message"="Add Script to Test", "Message Queue"=w473) -> ("error out"=w475:errorcluster[])  [unwired: 6 in, 1 out]
          }
        }
      }
      frame "----Cosmetics----" {
      }
      frame "Defer Panel Updates" {
        n195 = property class="VI"() -> (error out=w479:errorcluster, "Panel"=w480:refnum<vi>)  [unwired: 2 in, 1 out]
        n196 = property class="Pnl"(reference=w480, error in=w479, "DeferPanUpdts"=TRUE ("Defer Panel Updates")) -> ()  [unwired: 2 out]
      }
      frame "Update Panel" {
        n197 = property class="VI"() -> (error out=w483:errorcluster, "Panel"=w484:refnum<vi>)  [unwired: 2 in, 1 out]
        n198 = property class="Pnl"(reference=w484, error in=w483, "DeferPanUpdts"=FALSE ("Defer Panel Updates")) -> ()  [unwired: 2 out]
      }
    }
    n199 = call "Handle Error.vi"("ErrorArrayIn"=w40, "Message Queue"=w32) -> ("ErrorArrayOut"=w39:errorcluster[])  [unwired: 9 in]
  }
  n200 = call "cntlRefs.vi"() -> ("cntlRefs"=w14:T6)  [unwired: 10 in, 1 out]
  n201 = Bundle By Name(cluster=w14, "PluginTree"=w21, "pathUserfiles"=w7, "PluginTreeCaption"=w6, "PluginMgrQ"=w8) -> (w28:T6)
  n202 = call "cntlRefs.vi"("Set?"=TRUE, "cntlRefs"=w28) -> ("error out"=w11:errorcluster[])  [unwired: 8 in, 1 out]
  n203 = call "Enqueue.vi"("ErrorArray"=w11, "Message"="Plugin Manager Loaded") -> ("ErrorArray"=w10:errorcluster[])  [unwired: 9 in]
  n204 = while {
    tunnel: w31 -> [w493]
    shift-right: [w491] -> w24
    shift-left: w9 -> [w492]
    tunnel: w8 -> [w487]
    tunnel: w10 -> [_]
    tunnel: [w486] -> w5
    stop <- w490 stop-if-true
    # "My Event Handler"
    n205 = control-ref of="Severity"() -> (w489:refnum<vi>)
    n206 = event shown="[18] \"btnScriptHelper\": Value Change" {
      selector: w493 -> [_ _ _ _ _ _ _ _ _ _ _ _ _ _ _ _ _ _ _]
      dyn-events: [_ _ _ _ _ _ _ _ _ _ _ _ _ _ _ _ _ _ _] -> w486
      timeout: _ -> [_ _ _ _ _ _ _ _ _ _ _ _ _ _ _ _ _ _ _]
      tunnel: w492 -> [w500 w504 w509 _ _ _ w548 w552 w559 _ w565 w577 w580 w587 w594 _ w608 w649 _]
      tunnel: [w499 w503 w508 w513 _ w534 w547 w550 w558 _ w564 w576 w582 w589 w596 w597 w607 w648 _] -> w488
      tunnel: [TRUE ("Priority (F)") _ w507 _ _ _ _ _ _ TRUE ("Priority (F)") _ _ _ _ _ _ _ _ _] -> w490
      tunnel: w489 -> [_ _ _ _ _ _ _ _ _ _ _ _ _ _ _ _ _ _ _]
      tunnel: w487 -> [w494 _ w506 w514 _ w536 w545 w549 w556 _ w566 w578 w581 w588 w595 _ w606 w647 _]
      event Panel Close? {
        # "Stops the Framework and sends a message to the queued message handler to stop."
        n207 = event-data() -> ()  [unwired: 1 in, 4 out]
        n208 = call "Enqueue Message (Single).vi"("Priority Message? (F)"=TRUE ("Priority (F)"), "error in (no error)"=w500, "Message"="Stop", "Message Queue"=w494) -> ("error out"=w499:errorcluster[])  [unwired: 6 in, 1 out]
        n209 = event-data("Discard?"=TRUE) -> ()  [unwired: 1 in, 1 out]
      }
      event "Create Error (Test AutoTimeout)": Value Change {
        n210 = event-data() -> ()  [unwired: 1 in, 1 out]
        n211 = call <userlib>:"AddError.vi"("Severity"="Severity", "Priority"="Priority", "ErrorArray In"=w504, "error in (no error)"="Error In 2") -> ("ErrorArray Out"=w503:errorcluster[])  [unwired: 6 in, 1 out]
      }
      event User Event {
        w507 = TRUE ("Priority (F)")
        # "Queued Message Handler stops for any reason this top loop needs to also stop or an external stop call."
        n212 = event-data() -> ()  [unwired: 1 in, 1 out]
        n213 = call "Enqueue Message (Single).vi"("Priority Message? (F)"=w507, "error in (no error)"=w509, "Message"="Stop", "Message Queue"=w506) -> ("error out"=w508:errorcluster[])  [unwired: 6 in, 1 out]
      }
      event "btnNewScript": Value Change {
        n214 = event-data() -> ()  [unwired: 1 in, 1 out]
        n215 = call "cntlRefs.vi"() -> ("cntlRefs"=w515:T6)  [unwired: 10 in, 1 out]
        n216 = Unbundle By Name(w515) -> ("PluginTree"=w516:refnum<vi>)
        n217 = property class="Tree (strict)"(reference=w516) -> ("Value"=w511:string)  [unwired: 1 in, 2 out]
        n218 = call-poly "Enqueue Message.vi"("Message Data"=w511, "Message"="Create New Script", "Message Queue"=w514) -> ("error out"=w513:errorcluster[])  [unwired: 7 in, 1 out]
      }
      event "PluginTree": Value Change {
        n219 = event-data() -> ("NewVal"=w521:string)  [unwired: 1 in]
        n220 = call "Decode Plugin Tree Tag.vi"("Tag"=w521) -> ("Plugin Tree Tag"=w523:T8)  [unwired: 9 in, 1 out]
        n221 = Unbundle By Name(w523) -> ("ItemType"=w522:T5, "Script"=w520:string[])
        n222 = case shown="\"INI File\"" w522 {
          tunnel: w521 -> [_ _ _]
          tunnel: [T4."Disabled and Grayed Out" ("Disabled") T4."Enabled" ("Disabled") T4."Disabled and Grayed Out" ("Disabled")] -> w518
          tunnel: w520 -> [_ _ w532]
          tunnel: [_ _ w529] -> w519
          tunnel: [T4."Disabled and Grayed Out" ("Disabled") T4."Disabled and Grayed Out" ("Disabled") T4."Enabled" ("Disabled")] -> w517
          frame "Plugin", Default {
          }
          frame "INI File" {
          }
          frame "INI Script" {
            n223 = Array To Spreadsheet String(delimiter (Tab)="\n", array=w532, 3:"%s" ("format string")) -> (spreadsheet string=w529:string)
          }
        }
        n224 = local write "PluginScript"(w519) -> ()
        n225 = property on="btnAddToTest" class="Bool"("DisabledEnum"=w517) -> ()  [unwired: 2 in, 2 out]
        n226 = property on="btnConfig" class="Bool"("DisabledEnum"=w518) -> ()  [unwired: 2 in, 2 out]
        n227 = property on="btnNewScript" class="Bool"("DisabledEnum"=w518) -> ()  [unwired: 2 in, 2 out]
        n228 = property on="btnRunModule" class="Bool"("DisabledEnum"=w518) -> ()  [unwired: 2 in, 2 out]
        n229 = property on="btnDeleteScript" class="Bool"("DisabledEnum"=w517) -> ()  [unwired: 2 in, 2 out]
        n230 = property on="btnScriptHelper" class="Bool"("DisabledEnum"=w517) -> ()  [unwired: 2 in, 2 out]
        n231 = property on="btnRunScript" class="Bool"("DisabledEnum"=w517) -> ()  [unwired: 2 in, 2 out]
      }
      event "PluginScript": Value Change {
        n232 = event-data() -> ("NewVal"=w541:string)  [unwired: 1 in]
        n233 = call "cntlRefs.vi"() -> ("cntlRefs"=w538:T6)  [unwired: 10 in, 1 out]
        n234 = Unbundle By Name(w538) -> ("PluginTree"=w539:refnum<vi>)
        n235 = local read "OrigPluginTreeTags"() -> (w540:string[])
        n236 = call "Update Plugin Tree with New Script Value.vi"("New Script"=w541, "OrigPluginTreeTags"=w540, "TreeControl in"=w539) -> ("Save State"=w535:bool)  [unwired: 6 in, 2 out]
        n237 = call-poly "Enqueue Message.vi"("Message Data"=w535, "Message"="Plugin Tree Save State", "Message Queue"=w536) -> ("error out"=w534:errorcluster[])  [unwired: 7 in, 1 out]
      }
      event "btnConfig": Value Change {
        n238 = event-data() -> ()  [unwired: 1 in, 1 out]
        n239 = call "cntlRefs.vi"() -> ("cntlRefs"=w544:T6)  [unwired: 10 in, 1 out]
        n240 = Unbundle By Name(w544) -> ("PluginTree"=w543:refnum<vi>)
        n241 = property class="Tree (strict)"(reference=w543) -> ("Value"=w542:string)  [unwired: 1 in, 2 out]
        n242 = call-poly "Enqueue Message.vi"("error in (no error)"=w548, "Message Data"=w542, "Message"="OpenPrefDialog", "Message Queue"=w545) -> ("error out"=w547:errorcluster[])  [unwired: 6 in, 1 out]
      }
      event "btnSaveINIFiles": Value Change {
        n243 = event-data() -> ()  [unwired: 1 in, 1 out]
        n244 = call-poly "Enqueue Message.vi"("error in (no error)"=w552, "Message"="Save Scripts", "Message Queue"=w549) -> ("error out"=w550:errorcluster[])  [unwired: 7 in, 1 out]
      }
      event "btnAddToTest": Value Change {
        n245 = event-data() -> ()  [unwired: 1 in, 1 out]
        n246 = call "cntlRefs.vi"() -> ("cntlRefs"=w555:T6)  [unwired: 10 in, 1 out]
        n247 = Unbundle By Name(w555) -> ("PluginTree"=w554:refnum<vi>)
        n248 = property class="Tree (strict)"(reference=w554) -> ("Value"=w553:string)  [unwired: 1 in, 2 out]
        n249 = call-poly "Enqueue Message.vi"("error in (no error)"=w559, "Message Data"=w553, "Message"="Add Script to Test", "Message Queue"=w556) -> ("error out"=w558:errorcluster[])  [unwired: 6 in, 1 out]
      }
      event "Stop?": Value Change {
        n250 = event-data() -> ()  [unwired: 1 in, 1 out]
      }
      event "btnDeleteScript": Value Change {
        n251 = event-data() -> ()  [unwired: 1 in, 1 out]
        n252 = Two Button Dialog(message="Are you sure you want to delete this script?", 2:"Delete Script" ("T button name (\"OK\")")) -> (T button?=w561:bool)  [unwired: 1 in]
        n253 = case shown="True" w561 {
          tunnel: w566 -> [_ w574]
          tunnel: w565 -> [w567 w573]
          tunnel: [w567 w571] -> w564
          frame False {
          }
          frame True {
            n254 = call "cntlRefs.vi"() -> ("cntlRefs"=w570:T6)  [unwired: 10 in, 1 out]
            n255 = Unbundle By Name(w570) -> ("PluginTree"=w569:refnum<vi>)
            n256 = property class="Tree (strict)"(reference=w569) -> ("Value"=w568:string)  [unwired: 1 in, 2 out]
            n257 = call "Enqueue Message (Single).vi"("error in (no error)"=w573, "Message Data"=w568, "Message"="Delete Script", "Message Queue"=w574) -> ("error out"=w571:errorcluster[])  [unwired: 6 in, 1 out]
          }
        }
      }
      event "btnLoadUserFiles": Value Change {
        n258 = event-data() -> ()  [unwired: 1 in, 1 out]
        n259 = call "Enqueue Message (Single).vi"("error in (no error)"=w577, "Message"="Load Different Plugin Folder", "Message Queue"=w578) -> ("error out"=w576:errorcluster[])  [unwired: 7 in, 1 out]
      }
      event "btnRefresh": Value Change {
        n260 = event-data() -> ()  [unwired: 1 in, 1 out]
        n261 = call "Enqueue Message (Single).vi"("error in (no error)"=w580, "Message"="Refresh Tree", "Message Queue"=w581) -> ("error out"=w582:errorcluster[])  [unwired: 7 in, 1 out]
      }
      event "btnRunModule": Value Change {
        n262 = event-data() -> ()  [unwired: 1 in, 1 out]
        n263 = call "cntlRefs.vi"() -> ("cntlRefs"=w585:T6)  [unwired: 10 in, 1 out]
        n264 = Unbundle By Name(w585) -> ("PluginTree"=w584:refnum<vi>)
        n265 = property class="Tree (strict)"(reference=w584) -> ("Value"=w583:string)  [unwired: 1 in, 2 out]
        n266 = call "Enqueue Message (Single).vi"("error in (no error)"=w587, "Message Data"=w583, "Message"="Run a Module", "Message Queue"=w588) -> ("error out"=w589:errorcluster[])  [unwired: 6 in, 1 out]
      }
      event "btnRunScript": Value Change {
        n267 = event-data() -> ()  [unwired: 1 in, 1 out]
        n268 = call "cntlRefs.vi"() -> ("cntlRefs"=w592:T6)  [unwired: 10 in, 1 out]
        n269 = Unbundle By Name(w592) -> ("PluginTree"=w591:refnum<vi>)
        n270 = property class="Tree (strict)"(reference=w591) -> ("Value"=w590:string)  [unwired: 1 in, 2 out]
        n271 = call "Enqueue Message (Single).vi"("error in (no error)"=w594, "Message Data"=w590, "Message"="Run a Script", "Message Queue"=w595) -> ("error out"=w596:errorcluster[])  [unwired: 6 in, 1 out]
      }
      event "PluginTree": Shortcut Menu Activation? {
        n272 = event-data() -> ("MenuRef"=w602:refnum<k9>, "CtlRef"=w601:refnum<vi>, "Coords"=w600:T12)  [unwired: 1 in]
        n273 = invoke class="Tree (strict)" method="Point To Row Column"(reference=w601, "Point"=w600) -> ("Tag"=w599:string)  [unwired: 6 in, 7 out]
        n274 = call "CreatePluginTreeShortcutMenu.vi"("Tag"=w599, "Menu in"=w602) -> ("error out"=w598:errorcluster)  [unwired: 9 in]
        n275 = call <userlib>:"AddError.vi"("error in (no error)"=w598) -> ("ErrorArray Out"=w597:errorcluster[])  [unwired: 9 in, 1 out]
        n276 = event-data() -> ()  [unwired: 2 in, 1 out]
      }
      event "PluginTree": Shortcut Menu Selection (User) {
        n277 = event-data() -> ("ItemTag"=w609:string, "CtlRef"=w605:refnum<vi>, "Coords"=w604:T12)  [unwired: 1 in]
        n278 = invoke class="Tree (strict)" method="Point To Row Column"(reference=w605, "Point"=w604) -> ("Tag"=w603:string)  [unwired: 6 in, 7 out]
        n279 = case shown="\"Open in Editor\"" w609 {
          tunnel: w608 -> [w610 w614 w619 w624 w629 w634 w639 w644]
          tunnel: [w610 w613 w618 w623 w628 w633 w638 w643] -> w607
          tunnel: w606 -> [_ w612 w617 w622 w627 w632 w637 w642]
          tunnel: w603 -> [_ w611 w616 w621 w626 w631 w636 w641]
          frame Default {
          }
          frame "Run Module" {
            n280 = call "Enqueue Message (Single).vi"("error in (no error)"=w614, "Message Data"=w611, "Message"="Run a Module", "Message Queue"=w612) -> ("error out"=w613:errorcluster[])  [unwired: 6 in, 1 out]
          }
          frame "Create New Script" {
            n281 = call "Enqueue Message (Single).vi"("error in (no error)"=w619, "Message Data"=w616, "Message"="Create New Script", "Message Queue"=w617) -> ("error out"=w618:errorcluster[])  [unwired: 6 in, 1 out]
          }
          frame "Edit Configuration" {
            n282 = call "Enqueue Message (Single).vi"("error in (no error)"=w624, "Message Data"=w621, "Message"="OpenPrefDialog", "Message Queue"=w622) -> ("error out"=w623:errorcluster[])  [unwired: 6 in, 1 out]
          }
          frame "Run Script" {
            n283 = call "Enqueue Message (Single).vi"("error in (no error)"=w629, "Message Data"=w626, "Message"="Run a Script", "Message Queue"=w627) -> ("error out"=w628:errorcluster[])  [unwired: 6 in, 1 out]
          }
          frame "Add Script to Test" {
            n284 = call "Enqueue Message (Single).vi"("error in (no error)"=w634, "Message Data"=w631, "Message"="Add Script to Test", "Message Queue"=w632) -> ("error out"=w633:errorcluster[])  [unwired: 6 in, 1 out]
          }
          frame "Delete Script" {
            n285 = call "Enqueue Message (Single).vi"("error in (no error)"=w639, "Message Data"=w636, "Message"="Delete Script", "Message Queue"=w637) -> ("error out"=w638:errorcluster[])  [unwired: 6 in, 1 out]
          }
          frame "Open in Editor" {
            n286 = call "Enqueue Message (Single).vi"("error in (no error)"=w644, "Message Data"=w641, "Message"="Open in Editor", "Message Queue"=w642) -> ("error out"=w643:errorcluster[])  [unwired: 6 in, 1 out]
          }
        }
      }
      event "PluginTree": Double Click {
        n287 = event-data() -> ("Tag"=w646:string)  [unwired: 1 in]
        n288 = case shown="Default" w646 {
          selector: w646 -> [w653 _]
          tunnel: w649 -> [w656 w665]
          tunnel: [w655 w665] -> w648
          tunnel: w647 -> [w654 _]
          frame Default {
            n289 = call "Decode Plugin Tree Tag.vi"("Tag"=w653) -> ("Plugin Tree Tag"=w652:T8)  [unwired: 9 in, 1 out]
            n290 = Unbundle By Name(w652) -> ("ItemType"=w651:T5)
            n291 = case shown="\"INI Script\"" w651 {
              tunnel: [_ "Run a Module" ("Message") "Run a Script" ("Message")] -> w650
              frame "Plugin", Default {
              }
              frame "INI File" {
              }
              frame "INI Script" {
              }
            }
            n292 = case shown="Default" w650 {
              selector: w650 -> [_ w658]
              tunnel: w656 -> [w657 w662]
              tunnel: [w657 w661] -> w655
              tunnel: w654 -> [_ w660]
              tunnel: w653 -> [_ w659]
              frame "" {
              }
              frame Default {
                n293 = call "Enqueue Message (Single).vi"("error in (no error)"=w662, "Message Data"=w659, "Message"=w658, "Message Queue"=w660) -> ("error out"=w661:errorcluster[])  [unwired: 6 in, 1 out]
              }
            }
          }
          frame "" {
          }
        }
      }
      event "btnScriptHelper": Value Change {
        n294 = event-data() -> ()  [unwired: 1 in, 1 out]
        n295 = call "cntlRefs.vi"() -> ("cntlRefs"=w678:T6)  [unwired: 10 in, 1 out]
        n296 = Unbundle By Name(w678) -> ("PluginTree"=w677:refnum<vi>)
        n297 = property class="Tree (strict)"(reference=w677) -> (error out=w673:errorcluster, "Value"=w669:string)  [unwired: 1 in, 1 out]
        n298 = vi-ref "ScriptHelper.vi"() -> (w676:refnum<vi>)
        n299 = invoke class="VI" method="FP.Open"(reference=w676, error in=w673, "Activate"=TRUE ("Activate?"), "State"=T11."Standard") -> (reference out=w672:refnum<vi>, error out=w671:errorcluster)  [unwired: 1 in, 3 out]
        n300 = invoke class="VI" method="Ctrl Val.Set"(reference=w672, error in=w671, "Control Name"="Tag", "Value"=w669) -> (reference out=w668:refnum<vi>, error out=w667:errorcluster)  [unwired: 1 in, 3 out]
        n301 = invoke class="VI" method="Run VI"(reference=w668, error in=w667, "Wait until done"=FALSE ("Wait Until Done")) -> ()  [unwired: 2 in, 5 out]
      }
    }
    n302 = call "Handle Error.vi"("ErrorArrayIn"=w488, "Message Queue"=w487) -> ("ErrorArrayOut"=w491:errorcluster[])  [unwired: 9 in]
  }
  n303 = Unregister For Events(event registration refnum=w5) -> (error out=w4:errorcluster)  [unwired: 1 in]
  n304 = call <userlib>:"AddError.vi"("Severity"="Fatal", "Priority"=u8 0, "ErrorArray In"=w24, "error in (no error)"=w4) -> ("ErrorArray Out"=w23:errorcluster[])  [unwired: 6 in, 1 out]
  n305 = Merge Errors(w23, w27, w9) -> (w3:errorcluster)
  n306 = flat-sequence {
    tunnel: w1 -> [w682]
    tunnel: w3 -> [w679]
    tunnel: [w679] -> w2
    frame #0 {
      n307 = Unbundle By Name(w682) -> ("PluginMgrDidStop"=w681:refnum<user-event>)
      n308 = Generate User Event(user event=w681, event data cluster=T13 {"Data"=variant} ("event data")) -> ()  [unwired: 2 in, 2 out]
    }
  }
  "Error Out" <- w2
